vi "readPosition.vi"(3 "error in (no error)":errorcluster, 4 "VISA resource name":refnum<visa-resource-name>) -> (0 "error out":errorcluster, 1 "position":dbl format="%#.3g", 2 "VISA resource name out":refnum<visa-resource-name>)   [LabVIEW 2020]
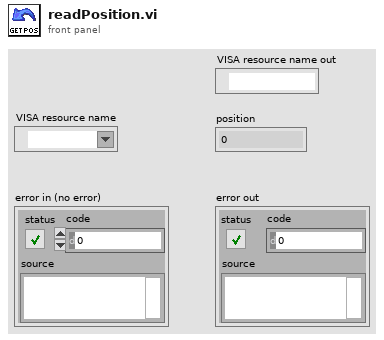
[diagram p1: front panel]
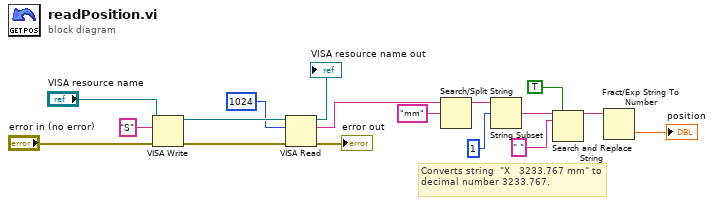
[diagram p0: block diagram]
diagram:
  # "Converts string  \"X   3233.767 mm\" to decimal number 3233.767."
  n1 = VISA Write(VISA resource name="VISA resource name", write buffer="S", error in (no error)="error in (no error)") -> (VISA resource name out=w16:refnum<visa-resource-name>, error out=w15:errorcluster)  [unwired: 1 out]
  n2 = VISA Read(VISA resource name=w16, byte count=u32 1024, error in (no error)=w15) -> (VISA resource name out=→"VISA resource name out":refnum<visa-resource-name>, read buffer=w2:string, error out=→"error out":errorcluster)  [unwired: 1 out]
  n3 = Search/Split String(string=w2, search string/char (-)="mm") -> (substring before match=w8:string)  [unwired: 1 in, 2 out]
  n4 = String Subset(string=w8, offset (0)=1) -> (substring=w7:string)  [unwired: 1 in]
  n5 = Search and Replace String(replace all?=TRUE ("replace all? (F)"), input string=w7, search string=" " ("search string/char (-)")) -> (result string=w4:string)  [unwired: 5 in, 3 out]
  n6 = Fract/Exp String To Number(string=w4) -> (number=→"position":dbl)  [unwired: 3 in, 1 out]
